vi "test Write and Read Boolean.vi"(8 "error in (no error)":errorcluster, 11 "TestCase in":refnum<class "Read Value Tests.lvclass">) -> (0 "error out":errorcluster, 3 "TestCase out":refnum<class "Read Value Tests.lvclass">)   [LabVIEW 2020, in "Memory Manager Tests.lvlib" / "Read Value Tests.lvclass"]
uses:
  Read Value Tests.lvclass
  Read Value Tests.lvclass/Read Value Tests.ctl
  Source/Classes/Pointer/Read Bool.vi
  <vilib>/addons/_JKI Toolkits/VI Tester/TestCase.llb/TestCase.lvclass
  Source/Classes/Pointer/Pointer.lvclass
  C:/Program Files (x86)/National Instruments/LabVIEW 2020/vi.lib/addons/_JKI Toolkits/VI Tester/TestCase.llb/TestCase.lvclass
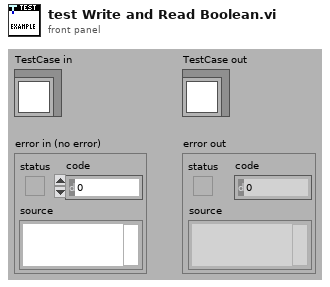
[diagram p1: front panel]
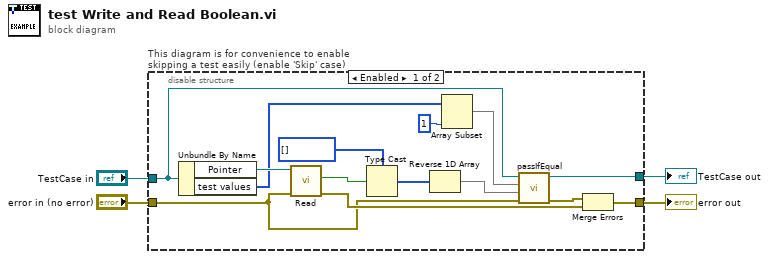
[diagram p0: block diagram]
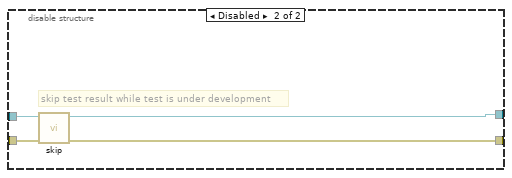
[diagram p2: hidden frame]
diagram:
  n1 = disable-structure "This diagram is for convenience to enable skipping a test easily (enable 'Skip' case)" shown="Enabled" {
    disable-tunnel: "TestCase in" -> [w10 w22]
    disable-tunnel: [w9 w20] -> w1
    disable-tunnel: [w7 w21] -> w3
    disable-tunnel: "error in (no error)" -> [w5 w19]
    frame Enabled {
      n2 = Unbundle By Name(w10) -> ("Pointer"=w14:refnum<class "Pointer.lvclass">, "test values"=w13:u8[])
      n3 = call-poly "Read.vi"("error in (no error)"=w5, "Pointer in"=w14) -> ("error out"=w6:errorcluster, "value out"=w17:bool)  [unwired: 6 in, 2 out]
      n4 = Type Cast(type=u8[] [] ("buffer in"), x=w17) -> (*(type *) &x=w18:u8[])
      n5 = Reverse 1D Array(array=w18) -> (reversed array=w11:u8[])
      n6 = Array Subset(array=w13, length=1) -> (w12:u8[])  [unwired: 1 in]
      n7 = call-dynamic "passIfEqual.vi"("error in (no error)"=w5, "y"=w11, "x"=w12, "TestCase in"=w10) -> ("error out"=w8:errorcluster, "TestCase out"=w9:refnum<class "Read Value Tests.lvclass">)  [unwired: 6 in]
      n8 = Merge Errors(w8, w6) -> (w7:errorcluster)
    }
    frame Disabled {
      # "skip test result while test is under development"
      n9 = call <vilib>:"skip.vi"("error in (no error)"=w19, "TestCase in"=w22) -> ("error out"=w21:errorcluster, "TestCase out"=w20:refnum<class "Read Value Tests.lvclass">)  [unwired: 8 in]
    }
  }
  "error out" <- w3
  "TestCase out" <- w1
